vi "Main.vi"() -> ()   [LabVIEW 2018]
doc: "Cet exemple de projet Mesure continue est basé sur le modèle Gestionnaire de messages dans une file d'attente.\n\nLa boucle de gestion d'événements génère des messages en fonction des actions sur l'interface utilisateur.\n\nLa boucle de gestion de messages traite les messages générés par la boucle de gestion d'événements ou par d'autres messages. Il y a aussi des sous-VIs de boucle de gestion de messages d'acquisition et d'enregistrement, ainsi qu'une boucle de mise à jour du graphe déroulant."
uses:
  Settings/Settings.ctl
  Acquisition/Hardware Configuration.ctl
  Acquisition/Signal Type.ctl
  Logging/Logging Configuration.ctl
  controls/UI Data.ctl
  controls/UI State.ctl
  support/Message Queue/Enqueue Message (Single).vi
  support/Message Queue/Enqueue Message (Array).vi
  <vilib>/Utility/error.llb/Error Cluster From Error Code.vi
  <vilib>/ErrorRing/Error Ring.xnode
  Acquisition/Acquisition.lvlib
  Logging/Logging.lvlib
  Settings/Settings.lvlib
  support/User Event - Stop/User Event - Stop.lvlib
  support/Message Queue/Message Queue.lvlib
  Settings/Settings Dialog.vi
panel:
  in  "Panneaux":enum32{"MAPA Tech"}(tab)
  out "Booléen":bool
  out "Longueur d'onde":dbl
  out "Puissance":dbl
  out "Puissance prédite":dbl
  out "Longueur d'onde":dbl(knob) scale=550.0..2550.0
  out "Puissance prédite":dbl(knob) scale=0.0..10.0
  out "Puissance":dbl(knob) scale=0.0..10.0
  in  "Param status":bool
  out "État":string
  in  "Quitter":bool
  in  "Arrêter":bool
  in  "Démarrer":bool
  in  "Paramètres":bool
  out "Données 2":cluster{dbl, dbl}(graph)
  out "Données":waveform(dbl)[](graph)
  out "Position X":dbl
  out "Position Y":dbl
  # "Position du faisceau"
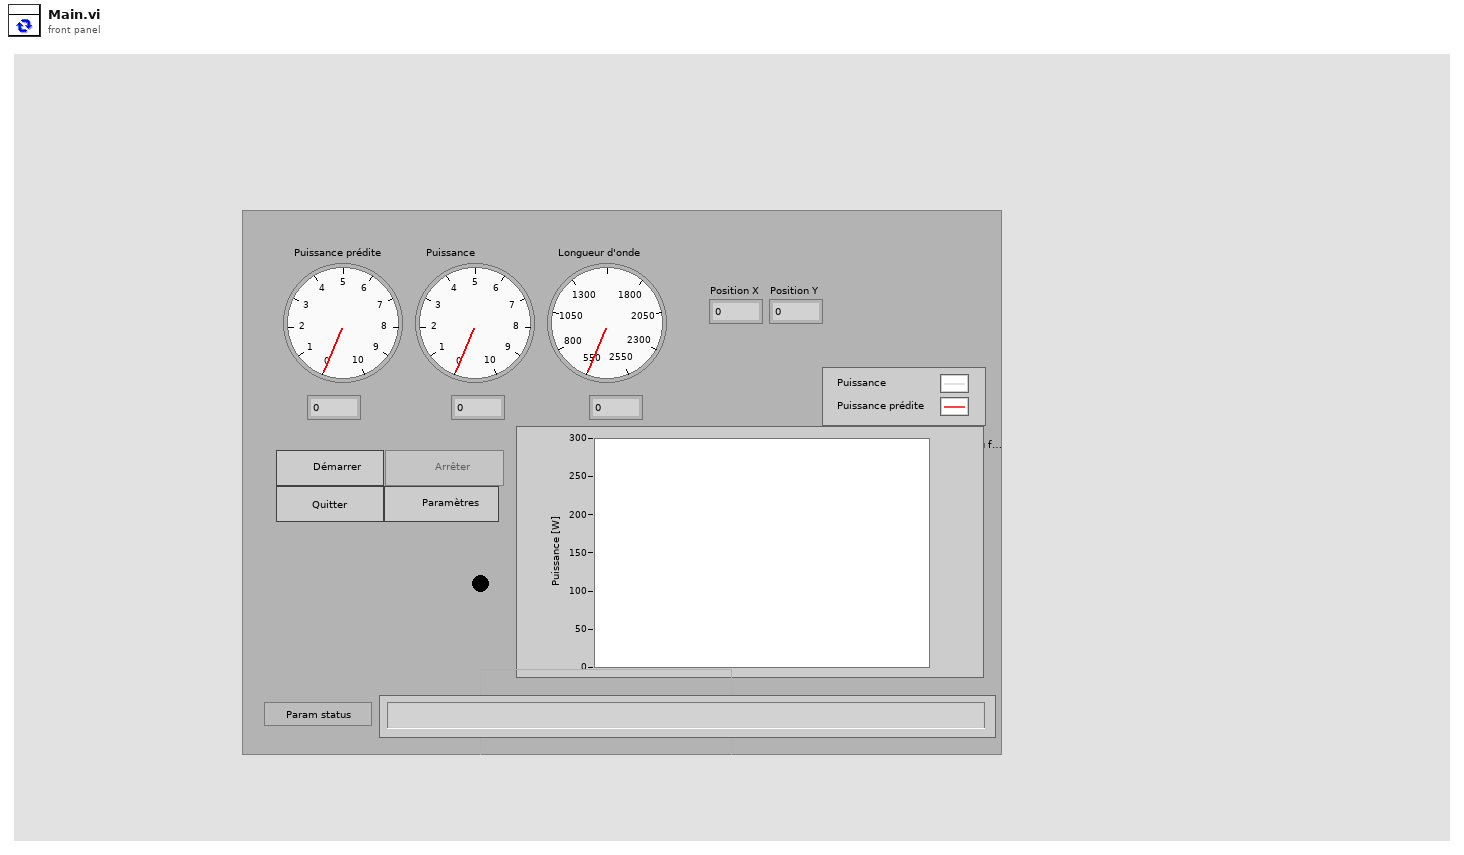
[diagram p1: front panel]
types:
  T1 = typedef "UI State.ctl" = enum16{"Idle", "Acquiring and Logging", "Waiting for Exit", "Waiting for Exit (Acq Stopped)", "Waiting for Exit (Log Stopped)", "Waiting for Stop", "Waiting for Stop (Acq Stopped)", "Waiting for Stop (Log Stopped)"}
  T2 = typedef "UI Data.ctl" = cluster{"Réf. de Démarrer":refnum<vi>, "Réf. d'Arrêter":refnum<vi>, "Réf. de Paramètres":refnum<vi>, "Réf. de Quitter":refnum<vi>, "Réf. d'état":refnum<vi>, "Réf. de données":refnum<vi>, "Ref. Moyennage sélectionneur":refnum<vi>, "Ref. Param status":refnum<vi>}
  T3 = typedef "Settings.lvlib/Settings.ctl" = cluster{"Configuration du matériel":T4, "Configuration de l'enregistrement":T6}
  T4 = typedef "Acquisition.lvlib/Hardware Configuration.ctl" = cluster{"Refnum de matériel <À remplacer>":string, "Type de signal <À remplacer>":T5, "Choix de la longueur d'onde":dbl, "Nom du périphérique":tag, "Choix mode":bool}
  T5 = typedef "Acquisition.lvlib/Signal Type.ctl" = enum16{"Sine Wave", "Square with Noise", "Signal triangulaire", "Simulation DAQ"}
  T6 = typedef "Logging.lvlib/Logging Configuration.ctl" = cluster{"Chemin de base du fichier journal":path, "Référence de fichier TDMS":refnum<k34>}
  T7 = cluster{"état":bool, "code":i32, "source":string}
  T8 = typedef "Message Queue.lvlib/All Message Queues.ctl" = cluster{"IU":refnum<queue>, "Acquisition":refnum<queue>, "Enregistrement":refnum<queue>}
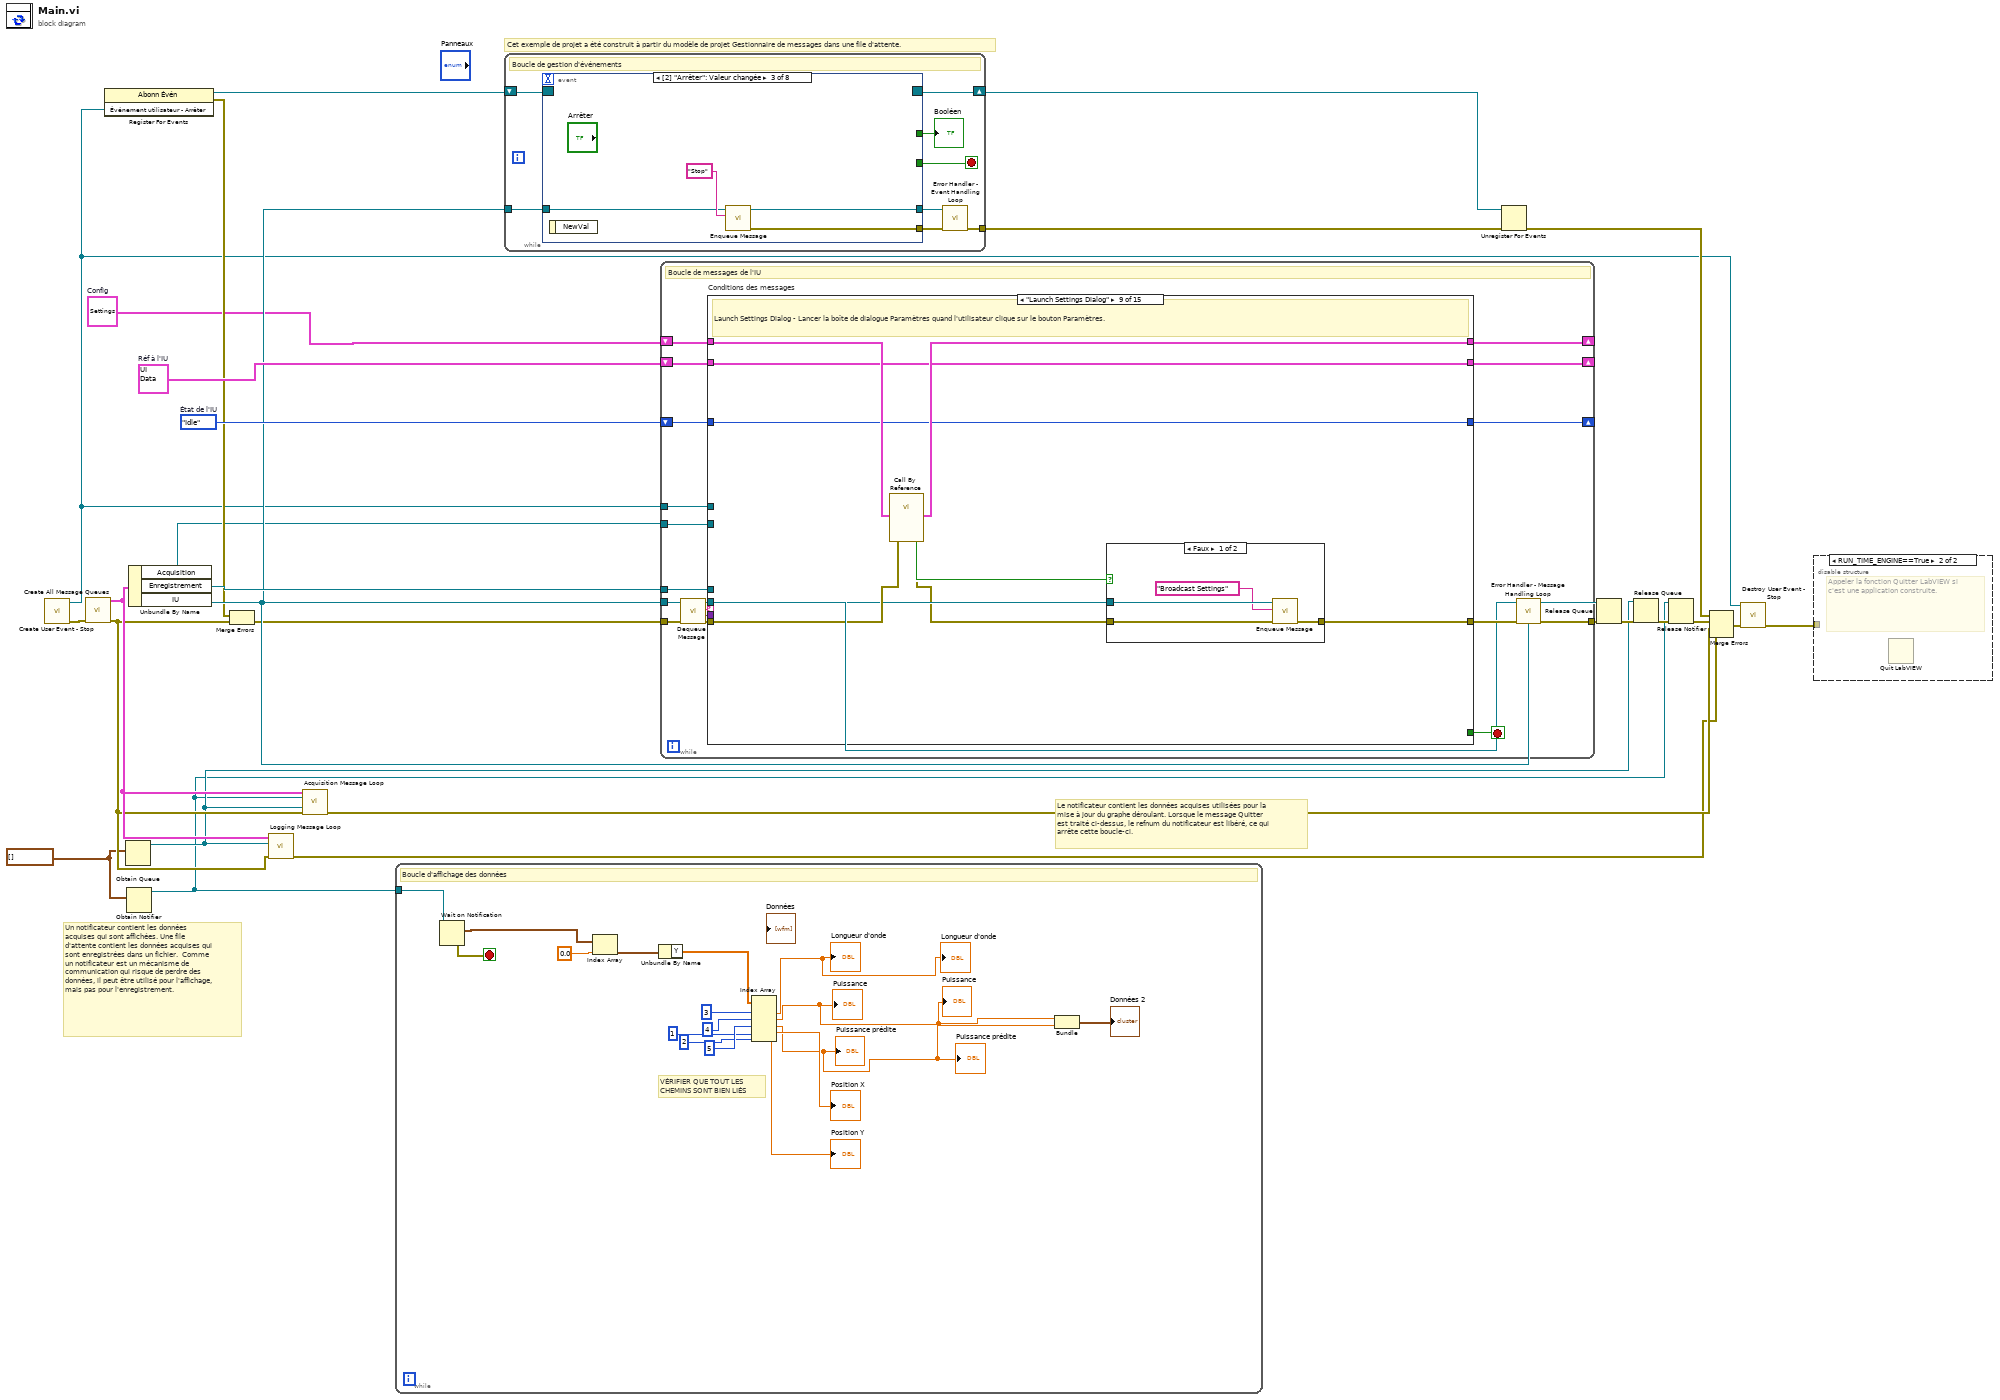
[diagram p0: block diagram]
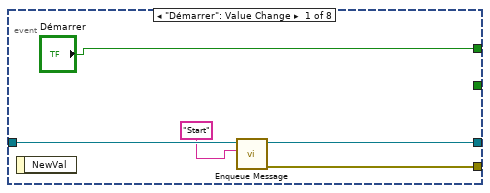
[diagram p3: hidden frame]
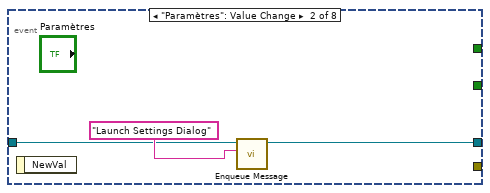
[diagram p4: hidden frame]
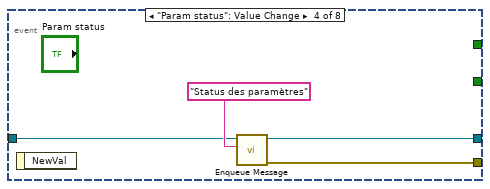
[diagram p5: hidden frame]
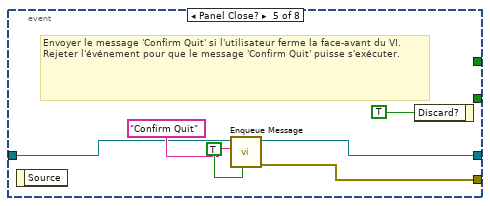
[diagram p6: hidden frame]
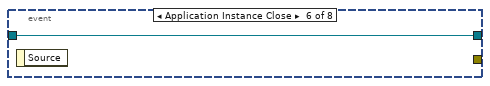
[diagram p7: hidden frame]
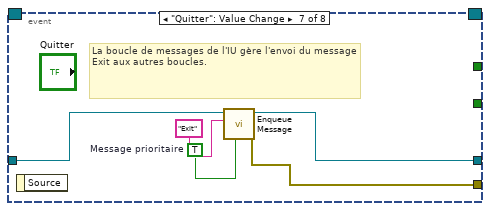
[diagram p8: hidden frame]
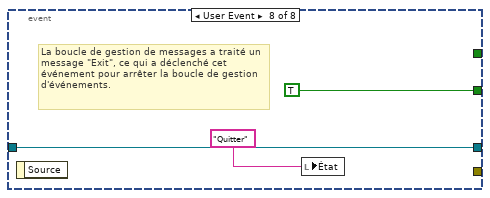
[diagram p9: hidden frame]
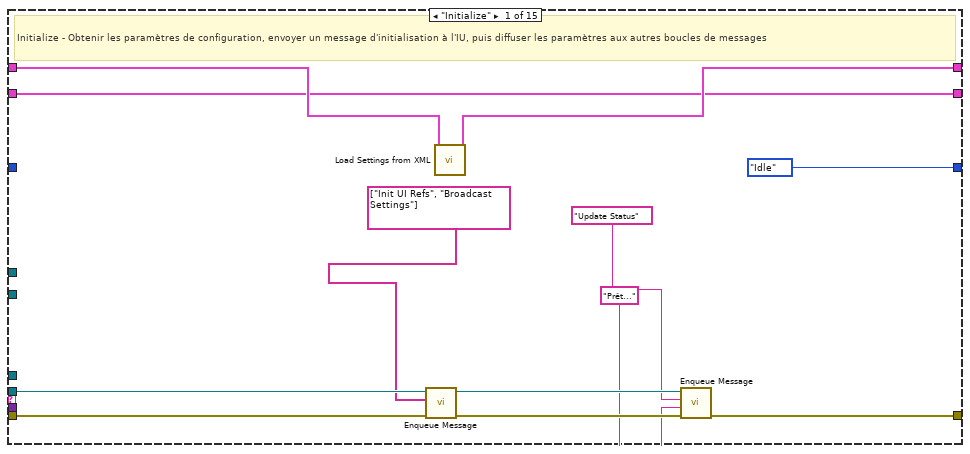
[diagram p10: hidden frame]
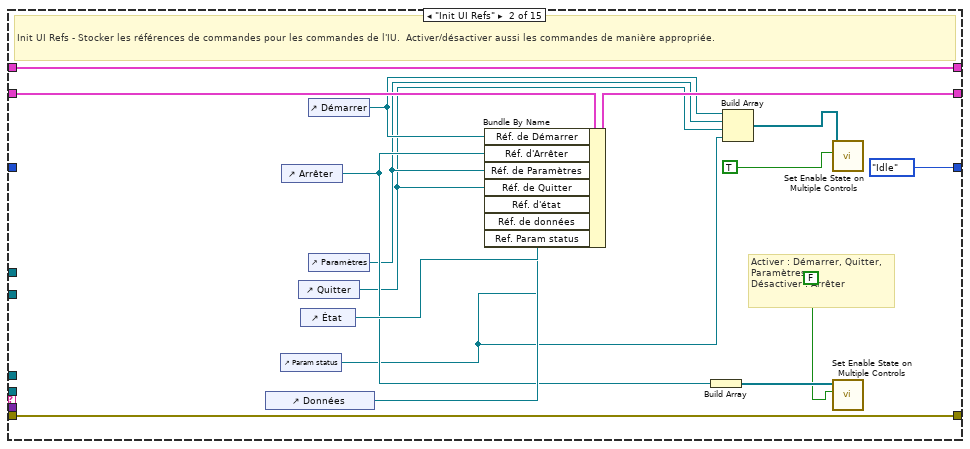
[diagram p11: hidden frame]
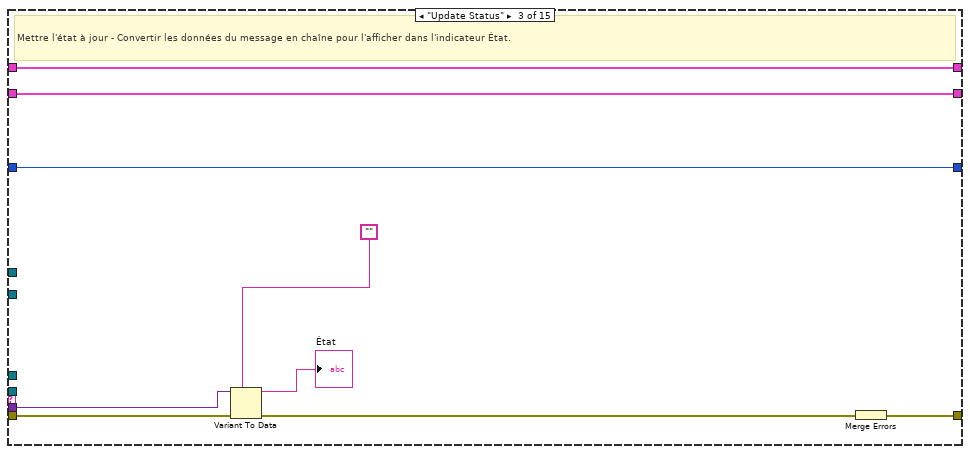
[diagram p12: hidden frame]
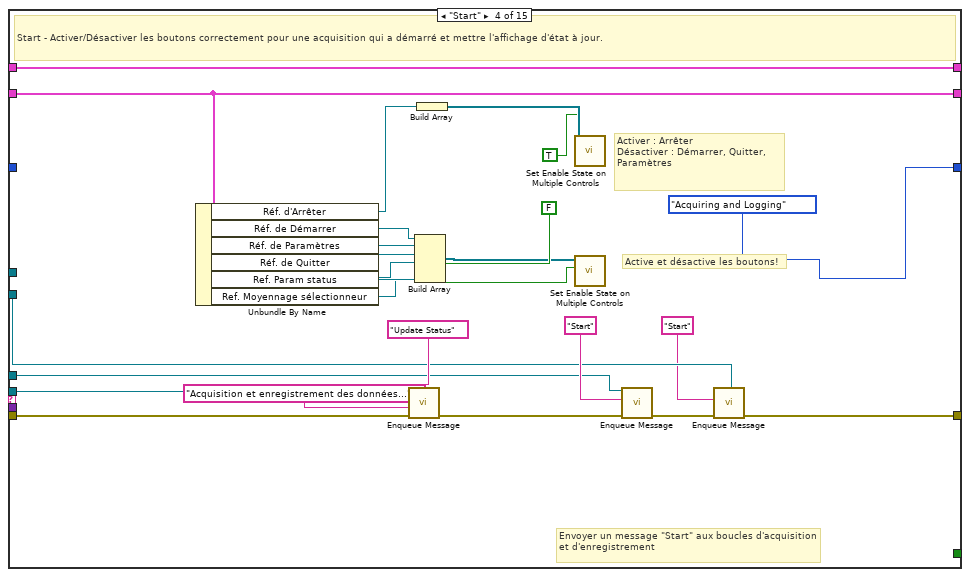
[diagram p13: hidden frame]
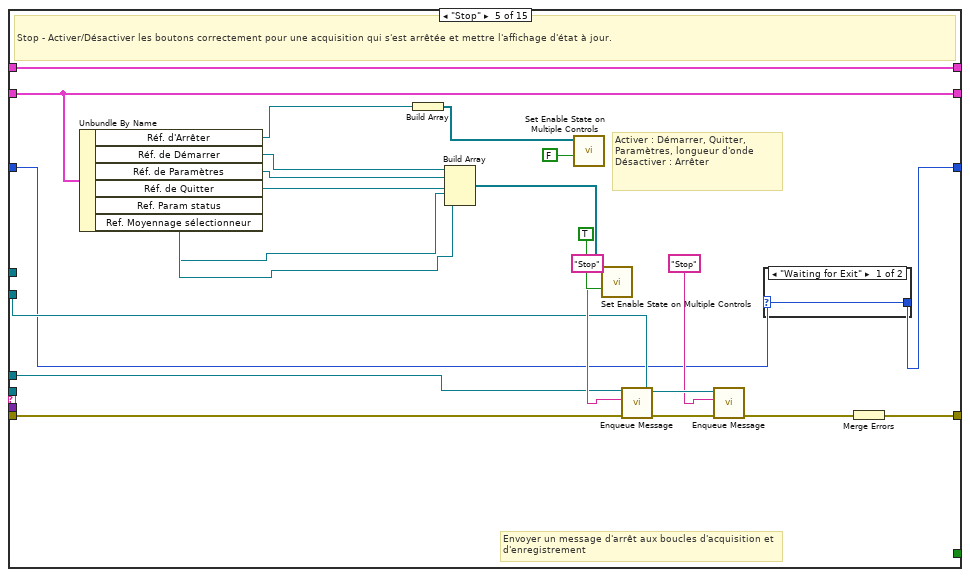
[diagram p14: hidden frame]
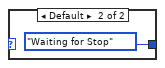
[diagram p15: hidden frame]
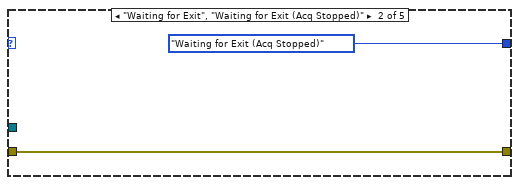
[diagram p17: hidden frame]
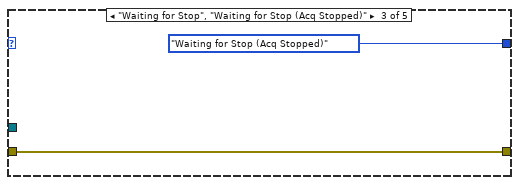
[diagram p18: hidden frame]
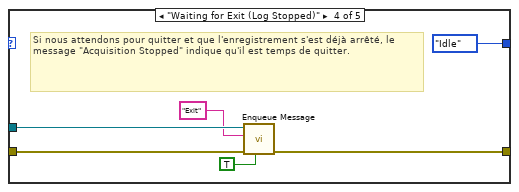
[diagram p19: hidden frame]
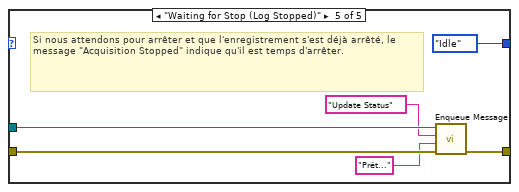
[diagram p20: hidden frame]
diagram:
  w16 = UI_State."Idle"  # État de l'IU
  w4 = waveform(dbl)[] []
  w18 = T2 {"Réf. de Démarrer"=refnum, "Réf. d'Arrêter"=refnum, "Réf. de Paramètres"=refnum, "Réf. de Quitter"=refnum, "Réf. d'état"=refnum, "Réf. de données"=refnum, "Ref. Moyennage sélectionneur"=refnum, "Ref. Param status"=refnum}  # Réf à l'IU
  w1 = T3 {"Configuration du matériel"={"Refnum de matériel <À remplacer>"="", "Type de signal <À remplacer>"=enum."Simulation DAQ", "Choix de la longueur d'onde"=500.0, "Nom du périphérique"="Dev1", "Choix mode"=FALSE}, "Configuration de l'enregistrement"={"Chemin de base du fichier journal"=path "", "Référence de fichier TDMS"=refnum}}  # Config
  # "Cet exemple de projet a été construit à partir du modèle de projet Gestionnaire de messages dans une file d'attente."
  # "Un notificateur contient les données acquises qui sont affichées. Une file d'attente contient les données acquises qui sont enregistrées dans un fichier.  Comme un notificateur est un mécanisme de communication qui risque de perdre des données, il peut être utilisé pour l'affichage, mais pas pour l'enregistrement."
  # "Le notificateur contient les données acquises utilisées pour la mise à jour du graphe déroulant. Lorsque le message Quitter est traité ci-dessus, le refnum du notificateur est libéré, ce qui arrête cette boucle-ci."
  n1 = call "Create User Event - Stop.vi"() -> ("error out"=w24:T7, "Événement utilisateur - Arrêter"=w5:refnum<user-event>)  [unwired: 10 in]
  n2 = call "Create All Message Queues.vi"("error in (no error)"=w24) -> ("error out"=w21:T7, "Files d'attente de messages en sortie"=w23:T8)  [unwired: 9 in]
  n3 = register-events(w5) -> (reference out=w9:refnum<event-registration>, error out=w7:errorcluster)  [unwired: 2 in]
  n4 = Obtain Queue(element data type=w4) -> (queue out=w3:refnum<queue>)  [unwired: 4 in, 2 out]
  n5 = Obtain Notifier(notification data type=w4) -> (notifier out=w2:refnum<notifier>)  [unwired: 3 in, 2 out]
  n6 = Unbundle By Name(w23) -> ("Acquisition"=w6:refnum<queue>, "Enregistrement"=w17:refnum<queue>, "IU"=w14:refnum<queue>)
  n7 = Merge Errors(w7, w21) -> (w8:errorcluster)
  n8 = call "Logging Message Loop.vi"("error in (no error)"=w21, "File d'attente de données"=w3, "Files d'attente de messages"=w23) -> ("error out"=w22:T7)  [unwired: 8 in]
  n9 = call "Acquisition Message Loop.vi"("Files d'attente de messages"=w23, "Notificateur de données"=w2, "File d'attente de données"=w3, "error in (no error)"=w21) -> ("error out"=w25:T7)  [unwired: 11 in]
  n10 = while "Data Display Loop" {
    tunnel: w2 -> [w43]
    stop <- w44 stop-if-true
    # "VÉRIFIER QUE TOUT LES \nCHEMINS SONT BIEN LIÉS"
    # "Boucle d'affichage des données"
    n11 = Wait on Notification(notifier=w43) -> (notification=w41:waveform(dbl)[], error out=w44:errorcluster)  [unwired: 3 in, 2 out]
    n12 = Index Array(array=w41, index=0.0) -> (element=w28:waveform(dbl))
    n13 = Unbundle By Name(w28) -> ("Y"=w40:dbl[])
    n14 = Index Array(array=w40, index #1=3, index #2=4, index #3=5 ("indice"), index #4=1 ("indice"), index #5=2 ("indice")) -> (element #1=→"Longueur d'onde" →"Longueur d'onde":dbl, element #2=w29:dbl, element #3=w30:dbl, element #4=→"Position X":dbl, element #5=→"Position Y":dbl)
    "Puissance" <- w29
    "Puissance prédite" <- w30
    "Puissance" <- w29
    "Puissance prédite" <- w30
    n15 = Bundle(w29, w30) -> (→"Données 2":cluster{dbl, dbl})  [unwired: 1 in]
  }
  n16 = while {
    tunnel: w14 -> [w51]
    tunnel: [w48] -> w26
    shift-right: [w50] -> w19
    shift-left: w9 -> [w52]
    stop <- w49 stop-if-true
    # "Boucle de gestion d'événements"
    n17 = event shown="[2] \"Arrêter\": Valeur changée" {
      selector: w52 -> [_ _ _ _ _ _ _ _]
      dyn-events: [_ _ _ _ _ _ _ _] -> w50
      timeout: _ -> [_ _ _ _ _ _ _ _]
      tunnel: [_ _ _ _ _ _ _ TRUE ("Discard?")] -> w49
      tunnel: w51 -> [w57 w59 w63 w67 w72 w75 w77 w81]
      tunnel: [w55 _ w62 w66 w70 _ w80 _] -> w47
      tunnel: [w54 w58 w61 w65 w71 w75 w76 w81] -> w46
      tunnel: ["Démarrer" _ _ _ _ _ _ _] -> w45
      event "Démarrer": Value Change {
        n18 = event-data() -> ()  [unwired: 1 in, 1 out]
        n19 = call-poly "Enqueue Message.vi"("Message"="Start", "File d'attente de messages"=w57) -> ("error out"=w55:T7, "File d'attente de message dup."=w54:refnum<queue>)  [unwired: 8 in]
      }
      event "Paramètres": Value Change {
        n20 = event-data() -> ()  [unwired: 1 in, 1 out]
        n21 = call-poly "Enqueue Message.vi"("Message"="Launch Settings Dialog", "File d'attente de messages"=w59) -> ("File d'attente de message dup."=w58:refnum<queue>)  [unwired: 8 in, 1 out]
      }
      event "Arrêter": Value Change {
        n22 = event-data() -> ()  [unwired: 1 in, 1 out]
        n23 = call-poly "Enqueue Message.vi"("Message"="Stop", "File d'attente de messages"=w63) -> ("error out"=w62:T7, "File d'attente de message dup."=w61:refnum<queue>)  [unwired: 8 in]
      }
      event "Param status": Value Change {
        n24 = event-data() -> ()  [unwired: 1 in, 1 out]
        n25 = call-poly "Enqueue Message.vi"("Message"="Status des paramètres", "File d'attente de messages"=w67) -> ("error out"=w66:T7, "File d'attente de message dup."=w65:refnum<queue>)  [unwired: 8 in]
      }
      event Panel Close? {
        # "Envoyer le message 'Confirm Quit' si l'utilisateur ferme la face-avant du VI. Rejeter l'événement pour que le message 'Confirm Quit' puisse s'exécuter."
        n26 = event-data() -> ()  [unwired: 1 in, 1 out]
        n27 = call-poly "Enqueue Message.vi"("Message prioritaire ? (F)"=TRUE ("Priority Message? (F)"), "Message"="Confirm Quit", "File d'attente de messages"=w72) -> ("error out"=w70:T7, "File d'attente de message dup."=w71:refnum<queue>)  [unwired: 7 in]
        n28 = event-data ("Event Filter Node")("Discard?"=TRUE) -> ()  [unwired: 1 in, 1 out]
      }
      event Application Instance Close {
        n29 = event-data() -> ()  [unwired: 1 in, 1 out]
      }
      event "Quitter": Value Change {
        w78 = TRUE  # Message prioritaire
        # "La boucle de messages de l'IU gère l'envoi du message Exit aux autres boucles."
        n30 = event-data() -> ()  [unwired: 1 in, 1 out]
        n31 = call-poly "Enqueue Message.vi"("Message prioritaire ? (F)"=w78, "Message"="Exit", "File d'attente de messages"=w77) -> ("error out"=w80:T7, "File d'attente de message dup."=w76:refnum<queue>)  [unwired: 7 in]
      }
      event User Event {
        # "La boucle de gestion de messages a traité un message \"Exit\", ce qui a déclenché cet événement pour arrêter la boucle de gestion d'événements."
        n32 = event-data() -> ()  [unwired: 1 in, 1 out]
        n33 = local write "État"("Quitter" ("Exit String")) -> ()
      }
    }
    "Booléen" <- w45
    n34 = call "Error Handler - Event Handling Loop.vi"("error in (no error)"=w47, "File d'attente de messages"=w46) -> ("erreur en entrée dup."=w48:T7)  [unwired: 8 in, 1 out]
  }
  n35 = while {
    tunnel: w14 -> [w95]
    tunnel: w5 -> [w100]
    shift-right: [w94] -> _
    shift-left: w1 -> [w93]
    shift-right: [w91] -> _
    shift-left: w18 -> [w92]
    tunnel: w6 -> [w90]
    tunnel: w17 -> [w89]
    shift-right: [w84] -> _
    shift-left: w16 -> [w85]
    tunnel: w8 -> [w99]
    tunnel: [w88] -> w27
    stop <- w101 stop-if-true
    # "Boucle de messages de l'IU"
    n36 = call "Dequeue Message.vi"("error in (no error)"=w99, "File d'attente de messages"=w95) -> ("error out"=w98:T7, "Données de message"=w96:variant, "Message"=w97:string, "File d'attente de message dup."=w86:refnum<queue>)  [unwired: 6 in]
    n37 = case "Conditions des messages" shown="\"Launch Settings Dialog\"" w97 {
      selector: w97 -> [_ _ _ _ _ _ _ _ _ _ _ _ _ _ w339]
      tunnel: w86 -> [w105 _ _ w162 _ w189 w214 _ w254 _ w275 _ _ w326 _]
      tunnel: w98 -> [w104 w129 w137 w161 w183 w190 w215 w242 w256 w263 w274 w303 w320 w330 _]
      tunnel: [w109 w129 w138 w148 w184 w187 w212 w248 w249 w266 w273 w313 w319 w329 w338] -> w87
      tunnel: [_ _ _ _ _ _ _ _ _ _ _ TRUE _ _ _] -> w101
      tunnel: w96 -> [_ _ w136 _ _ _ _ _ _ w267 _ w301 _ _ _]
      tunnel: w100 -> [_ _ _ _ _ _ _ _ _ _ _ w314 _ _ _]
      tunnel: [w112 w128 w132 w160 w182 w193 w218 w246 w253 w271 w278 w312 w318 w324 w342] -> w94
      tunnel: w93 -> [w113 w128 w132 w160 w182 w193 w218 w246 w257 w271 w278 w312 w318 w324 w342]
      tunnel: w92 -> [w106 w127 w131 w157 w181 w192 w217 w241 w251 w270 w277 w311 w317 w328 w341]
      tunnel: [w106 w124 w131 w157 w181 w192 w217 w241 w251 w270 w277 w311 w317 w328 w341] -> w91
      tunnel: w90 -> [_ _ _ w147 w174 _ _ w240 _ _ _ w310 _ _ _]
      tunnel: w89 -> [_ _ _ w150 w177 _ _ w237 _ _ _ w309 _ _ _]
      tunnel: w85 -> [_ _ w130 _ w171 w191 w216 w239 w250 w265 w276 _ w316 _ w340]
      tunnel: [UI_State."Idle" ("UI State") UI_State."Idle" ("UI State") w130 UI_State."Acquiring and Logging" ("UI State") w172 w188 w213 w239 w250 w265 w272 UI_State."Idle" ("UI State") w316 UI_State."Acquiring and Logging" ("UI State") w340] -> w84
      frame "Initialize" {
        # "Initialize - Obtenir les paramètres de configuration, envoyer un message d'initialisation à l'IU, puis diffuser les paramètres aux autres boucles de messages"
        n38 = call-poly "Enqueue Message.vi"("error in (no error)"=w104, "Tableau de messages"=string[] ["Init UI Refs", "Broadcast Settings"], "File d'attente de messages"=w105) -> ("error out"=w111:T7, "File d'attente de message dup."=w110:refnum<queue>)  [unwired: 7 in]
        n39 = call "Load Settings from XML.vi"("Paramètres en entrée"=w113) -> ("Paramètres en sortie"=w112:T3)  [unwired: 9 in, 1 out]
        n40 = call-poly "Enqueue Message.vi"("error in (no error)"=w111, "Données de message"="Prêt..." ("Ready..."), "Message"="Update Status", "File d'attente de messages"=w110) -> ("error out"=w109:T7)  [unwired: 6 in, 1 out]
      }
      frame "Init UI Refs" {
        # "Activer : Démarrer, Quitter, Paramètres\nDésactiver : Arrêter"
        # "Init UI Refs - Stocker les références de commandes pour les commandes de l'IU.  Activer/désactiver aussi les commandes de manière appropriée."
        n41 = control-ref of="Données"() -> (w125:refnum<vi>)
        n42 = control-ref of="Param status"() -> (w114:refnum<vi>)
        n43 = control-ref of="Arrêter"() -> (w119:refnum<vi>)
        n44 = control-ref of="Quitter"() -> (w116:refnum<vi>)
        n45 = control-ref of="État"() -> (w126:refnum<vi>)
        n46 = control-ref of="Démarrer"() -> (w118:refnum<vi>)
        n47 = control-ref of="Paramètres"() -> (w117:refnum<vi>)
        n48 = Bundle By Name(cluster=w127, "Réf. de Démarrer"=w118, "Réf. d'Arrêter"=w119, "Réf. de Paramètres"=w117, "Réf. de Quitter"=w116, "Réf. d'état"=w126, "Réf. de données"=w125, "Ref. Param status"=w114) -> (w124:T2)
        n49 = Build Array(w119) -> (w121:refnum<vi>[])
        n50 = Build Array(w118, w117, w116, w114) -> (w122:refnum<vi>[])
        n51 = call "Set Enable State on Multiple Controls.vi"("Activé ?"=TRUE ("Enable?"), "Commandes"=w122) -> ()  [unwired: 10 in]
        n52 = call "Set Enable State on Multiple Controls.vi"("Activé ?"=FALSE ("Enable?"), "Commandes"=w121) -> ()  [unwired: 10 in]
      }
      frame "Update Status" {
        # "Mettre l'état à jour - Convertir les données du message en chaîne pour l'afficher dans l'indicateur État."
        n53 = Variant To Data(error in=w137, type="" ("Empty String Constant"), Variant=w136) -> (data=→"État":string, error out=w134:errorcluster)
        n54 = Merge Errors(w134) -> (w138:errorcluster)
      }
      frame "Start" {
        # "Active et désactive les boutons!"
        # "Envoyer un message \"Start\" aux boucles d'acquisition et d'enregistrement"
        # "Activer : Arrêter\nDésactiver : Démarrer, Quitter, Paramètres"
        # "Start - Activer/Désactiver les boutons correctement pour une acquisition qui a démarré et mettre l'affichage d'état à jour."
        n55 = Unbundle By Name(w157) -> ("Réf. d'Arrêter"=w139:refnum<vi>, "Réf. de Démarrer"=w140:refnum<vi>, "Réf. de Paramètres"=w141:refnum<vi>, "Réf. de Quitter"=w144:refnum<vi>, "Ref. Param status"=w143:refnum<vi>, "Ref. Moyennage sélectionneur"=w142:refnum<vi>)
        n56 = call-poly "Enqueue Message.vi"("error in (no error)"=w161, "Données de message"="Acquisition et enregistrement des données..." ("Acquiring and Logging..."), "Message"="Update Status", "File d'attente de messages"=w162) -> ("error out"=w152:T7)  [unwired: 6 in, 1 out]
        n57 = Build Array(w140, w141, w141, w144, w143, w142) -> (w155:refnum<vi>[])
        n58 = Build Array(w139) -> (w154:refnum<vi>[])
        n59 = call "Set Enable State on Multiple Controls.vi"("Activé ?"=TRUE ("Enable?"), "Commandes"=w154) -> ()  [unwired: 10 in]
        n60 = call "Set Enable State on Multiple Controls.vi"("Activé ?"=FALSE ("Enable?"), "Commandes"=w155) -> ()  [unwired: 10 in]
        n61 = call-poly "Enqueue Message.vi"("error in (no error)"=w152, "Message"="Start", "File d'attente de messages"=w150) -> ("error out"=w149:T7)  [unwired: 7 in, 1 out]
        n62 = call-poly "Enqueue Message.vi"("error in (no error)"=w149, "Message"="Start", "File d'attente de messages"=w147) -> ("error out"=w148:T7)  [unwired: 7 in, 1 out]
      }
      frame "Stop" {
        # "Envoyer un message d'arrêt aux boucles d'acquisition et d'enregistrement"
        # "Activer : Démarrer, Quitter, Paramètres, longueur d'onde\nDésactiver : Arrêter"
        # "Stop - Activer/Désactiver les boutons correctement pour une acquisition qui s'est arrêtée et mettre l'affichage d'état à jour."
        n63 = Unbundle By Name(w181) -> ("Réf. d'Arrêter"=w163:refnum<vi>, "Réf. de Démarrer"=w164:refnum<vi>, "Réf. de Paramètres"=w165:refnum<vi>, "Réf. de Quitter"=w166:refnum<vi>, "Ref. Param status"=w167:refnum<vi>, "Ref. Moyennage sélectionneur"=w168:refnum<vi>)
        n64 = Build Array(w163) -> (w169:refnum<vi>[])
        n65 = Build Array(w164, w165, w166, w167, w168) -> (w170:refnum<vi>[])
        n66 = call "Set Enable State on Multiple Controls.vi"("Activé ?"=FALSE ("Enable?"), "Commandes"=w169) -> ()  [unwired: 10 in]
        n67 = call "Set Enable State on Multiple Controls.vi"("Activé ?"=TRUE ("Enable?"), "Commandes"=w170) -> ()  [unwired: 10 in]
        n68 = call-poly "Enqueue Message.vi"("error in (no error)"=w183, "Message"="Stop", "File d'attente de messages"=w177) -> ("error out"=w176:T7)  [unwired: 7 in, 1 out]
        n69 = call-poly "Enqueue Message.vi"("error in (no error)"=w176, "Message"="Stop", "File d'attente de messages"=w174) -> ("error out"=w175:T7)  [unwired: 7 in, 1 out]
        n70 = case shown="\"Waiting for Exit\"" w171 {
          selector: w171 -> [w185 _]
          tunnel: [w185 UI_State."Waiting for Stop" ("UI State")] -> w172
          frame "Waiting for Exit" {
          }
          frame Default {
          }
        }
        n71 = Merge Errors(w175) -> (w184:errorcluster)
      }
      frame "Acquisition Stopped" {
        # "Logique déterminant quelle action entreprendre quand l'acquisition s'est arrêtée."
        n72 = case shown="Par défaut" w191 {
          selector: w191 -> [w195 _ _ _ _]
          tunnel: w190 -> [w194 w197 w199 w205 w211]
          tunnel: w189 -> [_ _ _ w203 w208]
          tunnel: [w195 UI_State."Waiting for Exit (Acq Stopped)" ("UI State") UI_State."Waiting for Stop (Acq Stopped)" ("UI State") UI_State."Idle" ("UI State") UI_State."Idle" ("UI State")] -> w188
          tunnel: [w194 w197 w199 w204 w209] -> w187
          frame Default {
          }
          frame "Waiting for Exit", "Waiting for Exit (Acq Stopped)" {
          }
          frame "Waiting for Stop", "Waiting for Stop (Acq Stopped)" {
          }
          frame "Waiting for Exit (Log Stopped)" {
            # "Si nous attendons pour quitter et que l'enregistrement s'est déjà arrêté, le message \"Acquisition Stopped\" indique qu'il est temps de quitter."
            n73 = call-poly "Enqueue Message.vi"("Message prioritaire ? (F)"=TRUE ("Priority Message? (F)"), "error in (no error)"=w205, "Message"="Exit", "File d'attente de messages"=w203) -> ("error out"=w204:T7)  [unwired: 6 in, 1 out]
          }
          frame "Waiting for Stop (Log Stopped)" {
            # "Si nous attendons pour arrêter et que l'enregistrement s'est déjà arrêté, le message \"Acquisition Stopped\" indique qu'il est temps d'arrêter."
            n74 = call-poly "Enqueue Message.vi"("error in (no error)"=w211, "Données de message"="Prêt..." ("Ready..."), "Message"="Update Status", "File d'attente de messages"=w208) -> ("error out"=w209:T7)  [unwired: 6 in, 1 out]
          }
        }
      }
      frame "Logging Stopped" {
        # "Logique déterminant quelle action entreprendre quand l'enregistrement s'est arrêté."
        n75 = case shown="\"Waiting for Stop (Acq Stopped)\"" w216 {
          selector: w216 -> [w220 _ _ _ _]
          tunnel: w215 -> [w219 w222 w224 w230 w233]
          tunnel: w214 -> [_ _ _ w228 w232]
          tunnel: [w220 UI_State."Waiting for Exit (Log Stopped)" ("UI State") UI_State."Waiting for Stop (Log Stopped)" ("UI State") UI_State."Idle" ("UI State") UI_State."Idle" ("UI State")] -> w213
          tunnel: [w219 w222 w224 w229 w231] -> w212
          frame Default {
          }
          frame "Waiting for Exit", "Waiting for Exit (Log Stopped)" {
          }
          frame "Waiting for Stop", "Waiting for Stop (Log Stopped)" {
          }
          frame "Waiting for Exit (Acq Stopped)" {
            # "Si nous attendons pour quitter et que l'acquisition s'est déjà arrêtée, le message \"Logging Stopped\" indique qu'il est temps de quitter."
            n76 = call-poly "Enqueue Message.vi"("Message prioritaire ? (F)"=TRUE ("Priority Message? (F)"), "error in (no error)"=w230, "Message"="Exit", "File d'attente de messages"=w228) -> ("error out"=w229:T7)  [unwired: 6 in, 1 out]
          }
          frame "Waiting for Stop (Acq Stopped)" {
            # "Si nous attendons pour arrêter et que l'acquisition s'est déjà arrêtée, le message \"Logging Stopped\" indique qu'il est temps d'arrêter."
            n77 = call-poly "Enqueue Message.vi"("error in (no error)"=w233, "Données de message"="Prêt..." ("Ready..."), "Message"="Update Status", "File d'attente de messages"=w232) -> ("error out"=w231:T7)  [unwired: 6 in, 1 out]
          }
        }
      }
      frame "Broadcast settings" {
        w238 = "Update Settings" ("Message")
        # "Broadcast settings - Envoyer le message 'Update Settings' aux boucles de messages d'enregistrement et d'acquisition."
        n78 = Unbundle By Name(w246) -> ("Configuration du matériel"=w245:T4, "Configuration de l'enregistrement"=w244:T6)
        n79 = call-poly "Enqueue Message.vi"("Données de message"=w245, "Message"=w238, "File d'attente de messages"=w240) -> ("error out"=w247:T7)  [unwired: 7 in, 1 out]
        n80 = call-poly "Enqueue Message.vi"("error in (no error)"=w247, "Données de message"=w244, "Message"=w238, "File d'attente de messages"=w237) -> ("error out"=w243:T7)  [unwired: 6 in, 1 out]
        n81 = Merge Errors(w243, w242) -> (w248:errorcluster)
      }
      frame "Launch Settings Dialog" {
        # "Launch Settings Dialog - Lancer la boîte de dialogue Paramètres quand l'utilisateur clique sur le bouton Paramètres."
        n82 = call-by-ref "?"("error in (no error)"=w256, "Paramètres en entrée"=w257) -> ("error out"=w252:T7, "Annulation ?"=w255:bool, "Paramètres en sortie"=w253:T3)  [unwired: 8 in, 3 out]
        n83 = case shown="Faux" w255 {
          tunnel: w254 -> [w261 _]
          tunnel: w252 -> [w260 w262]
          tunnel: [w259 w262] -> w249
          frame False {
            n84 = call-poly "Enqueue Message.vi"("error in (no error)"=w260, "Message"="Broadcast Settings", "File d'attente de messages"=w261) -> ("error out"=w259:T7)  [unwired: 7 in, 1 out]
          }
          frame True {
          }
        }
      }
      frame "Error" {
        # "Error - Afficher une boîte de dialogue d'erreur. Ce message est envoyé par les VIs \"Error Handler\" à la fin de l'exécution de chaque boucle de cette application."
        n85 = Variant To Data(error in=w263, type=errorcluster {"status"=FALSE, "code"=0, "source"=""} ("error constant"), Variant=w267) -> (data=w264:errorcluster, error out=w268:errorcluster)
        n86 = call <vilib>:"Simple Error Handler.vi"("error in (no error)"=w264) -> ()  [unwired: 4 in, 5 out]
        n87 = Merge Errors(w268) -> (w266:errorcluster)
      }
      frame "Confirm Quit" {
        # "Confirm Quit - Message qui confirme si l'utilisateur voulait vraiment quitter l'application."
        n88 = case shown="\"Acquiring and Logging\"" w276 {
          tunnel: w275 -> [w284 w288]
          tunnel: w274 -> [w283 w287]
          tunnel: [w282 w286] -> w273
          tunnel: [UI_State."Idle" ("UI State") w285] -> w272
          frame Default {
            # "Si 'Confirm Quit' survient alors que le système est inactif, le message de confirmation est inutile."
            n89 = call-poly "Enqueue Message.vi"("Message prioritaire ? (F)"=TRUE ("Priority Message? (F)"), "error in (no error)"=w283, "Message"="Exit", "File d'attente de messages"=w284) -> ("error out"=w282:T7)  [unwired: 6 in, 1 out]
          }
          frame "Acquiring and Logging" {
            n90 = Two Button Dialog(message="Voulez-vous vraiment quitter en cours d'acquisition ?" ("Confirm Quit Message"), 1:"Non" ("No"), 2:"Oui" ("Yes")) -> (T button?=w289:bool)
            n91 = case shown="Vrai" w289 {
              tunnel: w288 -> [_ w298]
              tunnel: w287 -> [w294 w299]
              tunnel: [w294 w297] -> w286
              tunnel: [UI_State."Acquiring and Logging" ("UI State") UI_State."Waiting for Exit" ("UI State")] -> w285
              frame False {
                # "L'utilisateur ne voulait pas quitter."
              }
              frame True {
                n92 = call-poly "Enqueue Message.vi"("error in (no error)"=w299, "Message"="Stop", "File d'attente de messages"=w298) -> ("error out"=w297:T7)  [unwired: 7 in, 1 out]
              }
            }
          }
        }
      }
      frame "Exit" {
        w305 = TRUE ("Priority Message? (F)")
        w306 = "Exit" ("Message")
        # "Afficher une boîte de dialogue d'erreur si 'Exit' a été appelé suite à une erreur."
        # "Arrêter le VI"
        # "Exit - Envoyer des messages Exit aux boucles d'acquisition et d'enregistrerment, et déclencher l'événement utilisateur pour arrêter la boucle de gestion d'événements."
        n93 = Variant To Data(type=errorcluster {"status"=FALSE, "code"=0, "source"=""} ("error constant"), Variant=w301) -> (data=w300:errorcluster)  [unwired: 1 in, 1 out]
        n94 = call <vilib>:"Simple Error Handler.vi"("error in (no error)"=w300) -> ()  [unwired: 4 in, 5 out]
        n95 = call-poly "Enqueue Message.vi"("Message prioritaire ? (F)"=w305, "error in (no error)"=w303, "Message"=w306, "File d'attente de messages"=w310) -> ("error out"=w307:T7)  [unwired: 6 in, 1 out]
        n96 = call-poly "Enqueue Message.vi"("Message prioritaire ? (F)"=w305, "error in (no error)"=w307, "Message"=w306, "File d'attente de messages"=w309) -> ("error out"=w304:T7)  [unwired: 6 in, 1 out]
        n97 = call "Fire User Event - Stop.vi"("error in (no error)"=w304, "Événement utilisateur - Arrêt"=w314) -> ("error out"=w313:T7)  [unwired: 9 in]
      }
      frame "---Copy This Frame---" {
        # "Dupliquez cette étape pour créer de nouveaux messages.  Changez ce commentaire dans l'étape dupliquée pour décrire ce message."
        n98 = Merge Errors(w320) -> (w319:errorcluster)
      }
      frame "Status des paramètres" {
        # "Dupliquez cette étape pour créer de nouveaux messages.  Changez ce commentaire dans l'étape dupliquée pour décrire ce message."
        n99 = Unbundle By Name(w324) -> ("Configuration du matériel.Choix mode"=w323:bool, "Configuration du matériel.Choix de la longueur d'onde"=w322:dbl)
        n100 = case shown="Vrai" w323 {
          tunnel: [w331 w336] -> w321
          tunnel: w322 -> [_ w337]
          frame False {
            n101 = Concatenate Strings ("Concaténer des chaînes")("Status: Mode automatique") -> (w331:string)
          }
          frame True {
            n102 = Number To Decimal String(number=w337) -> (decimal integer string=w334:string)  [unwired: 1 in]
            n103 = Concatenate Strings ("Concaténer des chaînes")("Status: Mode manuel et la longueur d'onde sélectionnée est ", w334, " nm.") -> (w336:string)
          }
        }
        n104 = Merge Errors(w330) -> (w329:errorcluster)
        n105 = call-poly "Enqueue Message.vi"("Données de message"=w321, "Message"="Update Status", "File d'attente de messages"=w326) -> ()  [unwired: 7 in, 2 out]
      }
      frame Default {
        # "La condition 'Par défaut' ne s'exécute que s'il y a un message qui n'est défini dans aucune des autres conditions.  Renvoyer une erreur de programmation."
        n106 = xnode ("Error Ring")("paramètre 0"=w339) -> ("sortie d'erreur"=w338:errorcluster)
      }
    }
    n107 = call "Error Handler - Message Handling Loop.vi"("error in (no error)"=w87, "File d'attente de messages"=w86) -> ("erreur en entrée dup."=w88:T7)  [unwired: 8 in, 1 out]
  }
  n108 = Unregister For Events(event registration refnum=w19, error in=w26) -> (error out=w20:errorcluster)
  n109 = Release Queue(queue=w14, error in (no error)=w27) -> (error out=w12:errorcluster)  [unwired: 1 in, 2 out]
  n110 = Release Queue(queue=w3, error in (no error)=w12) -> (error out=w11:errorcluster)  [unwired: 1 in, 2 out]
  n111 = Release Notifier(notifier=w2, error in (no error)=w11) -> (error out=w10:errorcluster)  [unwired: 1 in, 2 out]
  n112 = Merge Errors(w20, w10, w25, w22) -> (w15:errorcluster)
  n113 = call "Destroy User Event - Stop.vi"("error in (no error)"=w15, "Événement utilisateur - Arrêt"=w5) -> ("error out"=w13:T7)  [unwired: 9 in]
  n114 = disable-structure "Conditional Disable Structure" shown="RUN_TIME_ENGINE==True" {
    disable-tunnel: w13 -> [_ _]
    frame condition #0 (active) {
    }
    frame condition #1 {
      # "Appeler la fonction Quitter LabVIEW si c'est une application construite."
      n115 = Quit LabVIEW() -> ()  [unwired: 1 in]
    }
  }
